vi "Take and analyse picture.vi"(0 "Training image on/off":bool, 2 "Session Out in":T3, 3 "Refnum in":T1, 5 "error in (no error)":errorcluster) -> (9 "error out":errorcluster, 10 "output cluster":T2, 14 "Insect-data-array (out of range removed)":dbl[][](array[numeric]), 15 "Initial number of insects":i32, 16 "Number of objects":i32, 17 "Session Out out":T3, 18 "Tegne cirkel array":dbl[][](array[numeric]), 19 "Black image error":bool)   [LabVIEW 2022 SP3]
doc: "Collects an image and runs it throu the vision asistent. Then transforms output data to sutible outlets and formats."
uses:
  <vilib>/userdefined/High Color/IMAQdx.ctl
  <vilib>/vision/Image Controls.llb/IMAQ Image.ctl
  <vilib>/vision/NI_Vision_Development_Module.lvlib
  <vilib>/vision/driver/NI_Vision_Acquisition_Software.lvlib
panel:
  out "Camera feed":T1(plugin-control)
  in  "Boolean":bool
  out "Image from vision assistant 2":T1(plugin-control)
  out "T_and_A Stoped":bool
  out "Match Score (Color Matching 1)":i32[](array[numeric])
  out "Objects after sorting":string[][](array[string])
  out "Image from vision assistant":T1(plugin-control)
  in  "Stop program":bool
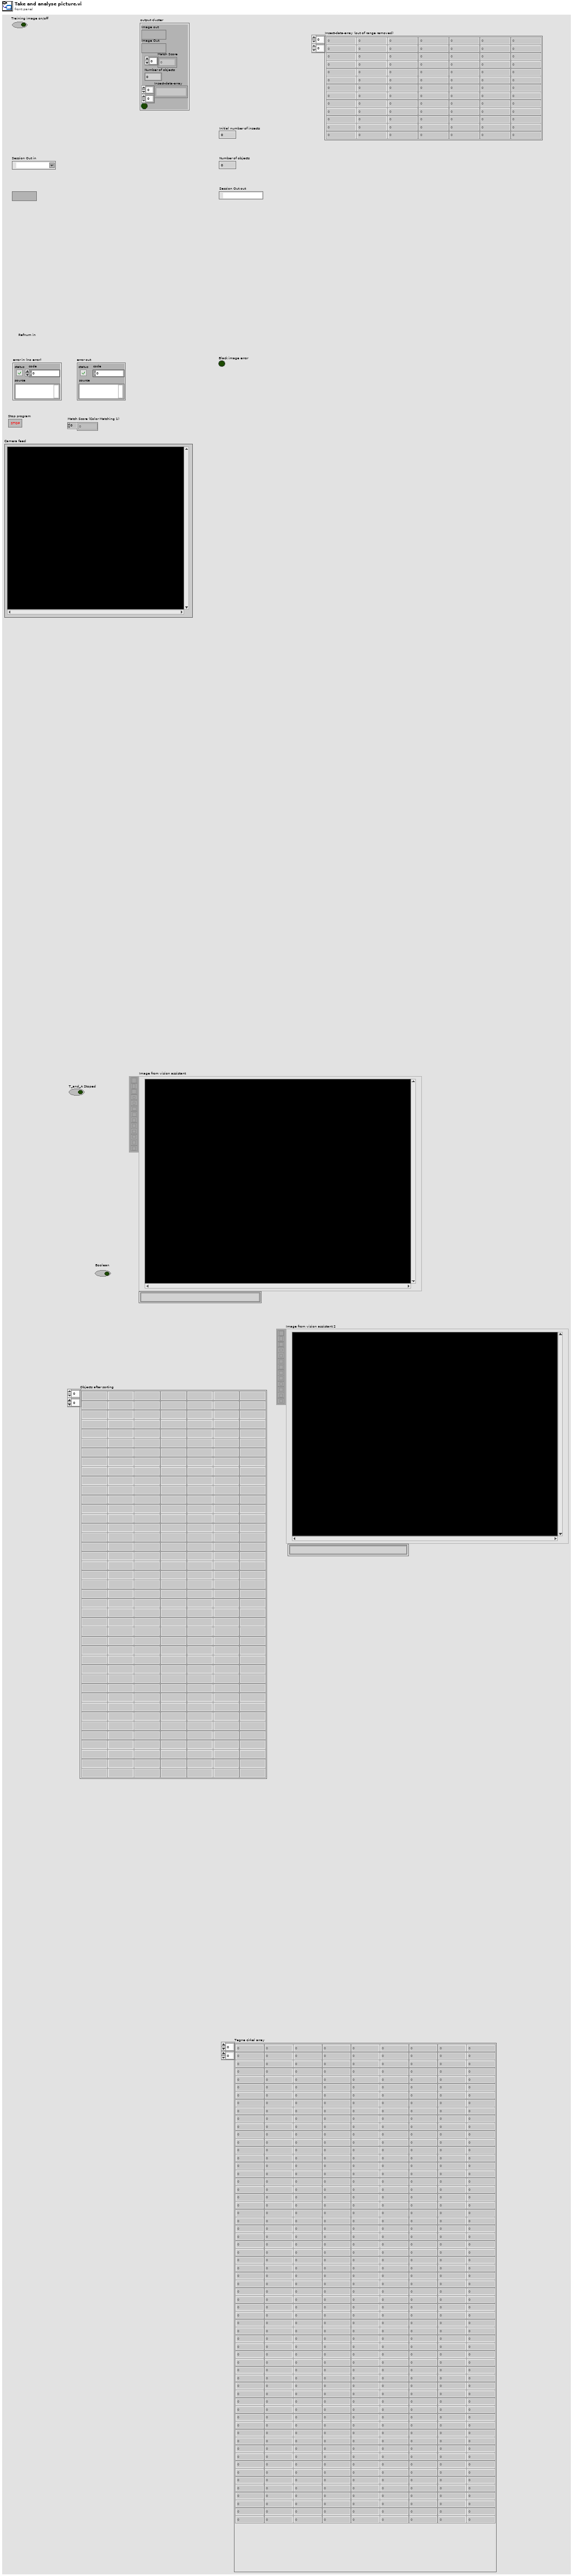
[diagram p1: front panel]
types:
  T1 = typedef "IMAQ Image.ctl" = refnum<image>
  T2 = cluster{"Image out":T1, "Image Out":T1, "Match Score":i32[], "Number of objects":i32, "Insect-data-array":string[][], bool}
  T3 = typedef "IMAQdx.ctl" = refnum<k21>
  T4 = cluster{"Measurement Parameter":i32, "Range Lower Value":dbl, "Range Upper Value":dbl, "Range":bool, "Measurement Type":bool}[]
  T5 = cluster{"Image out":T1, "Image Out":T1, "Match Score (Color Matching 1)":i32[], "Number of objects":i32, "Insect-data-array":string[][], bool}
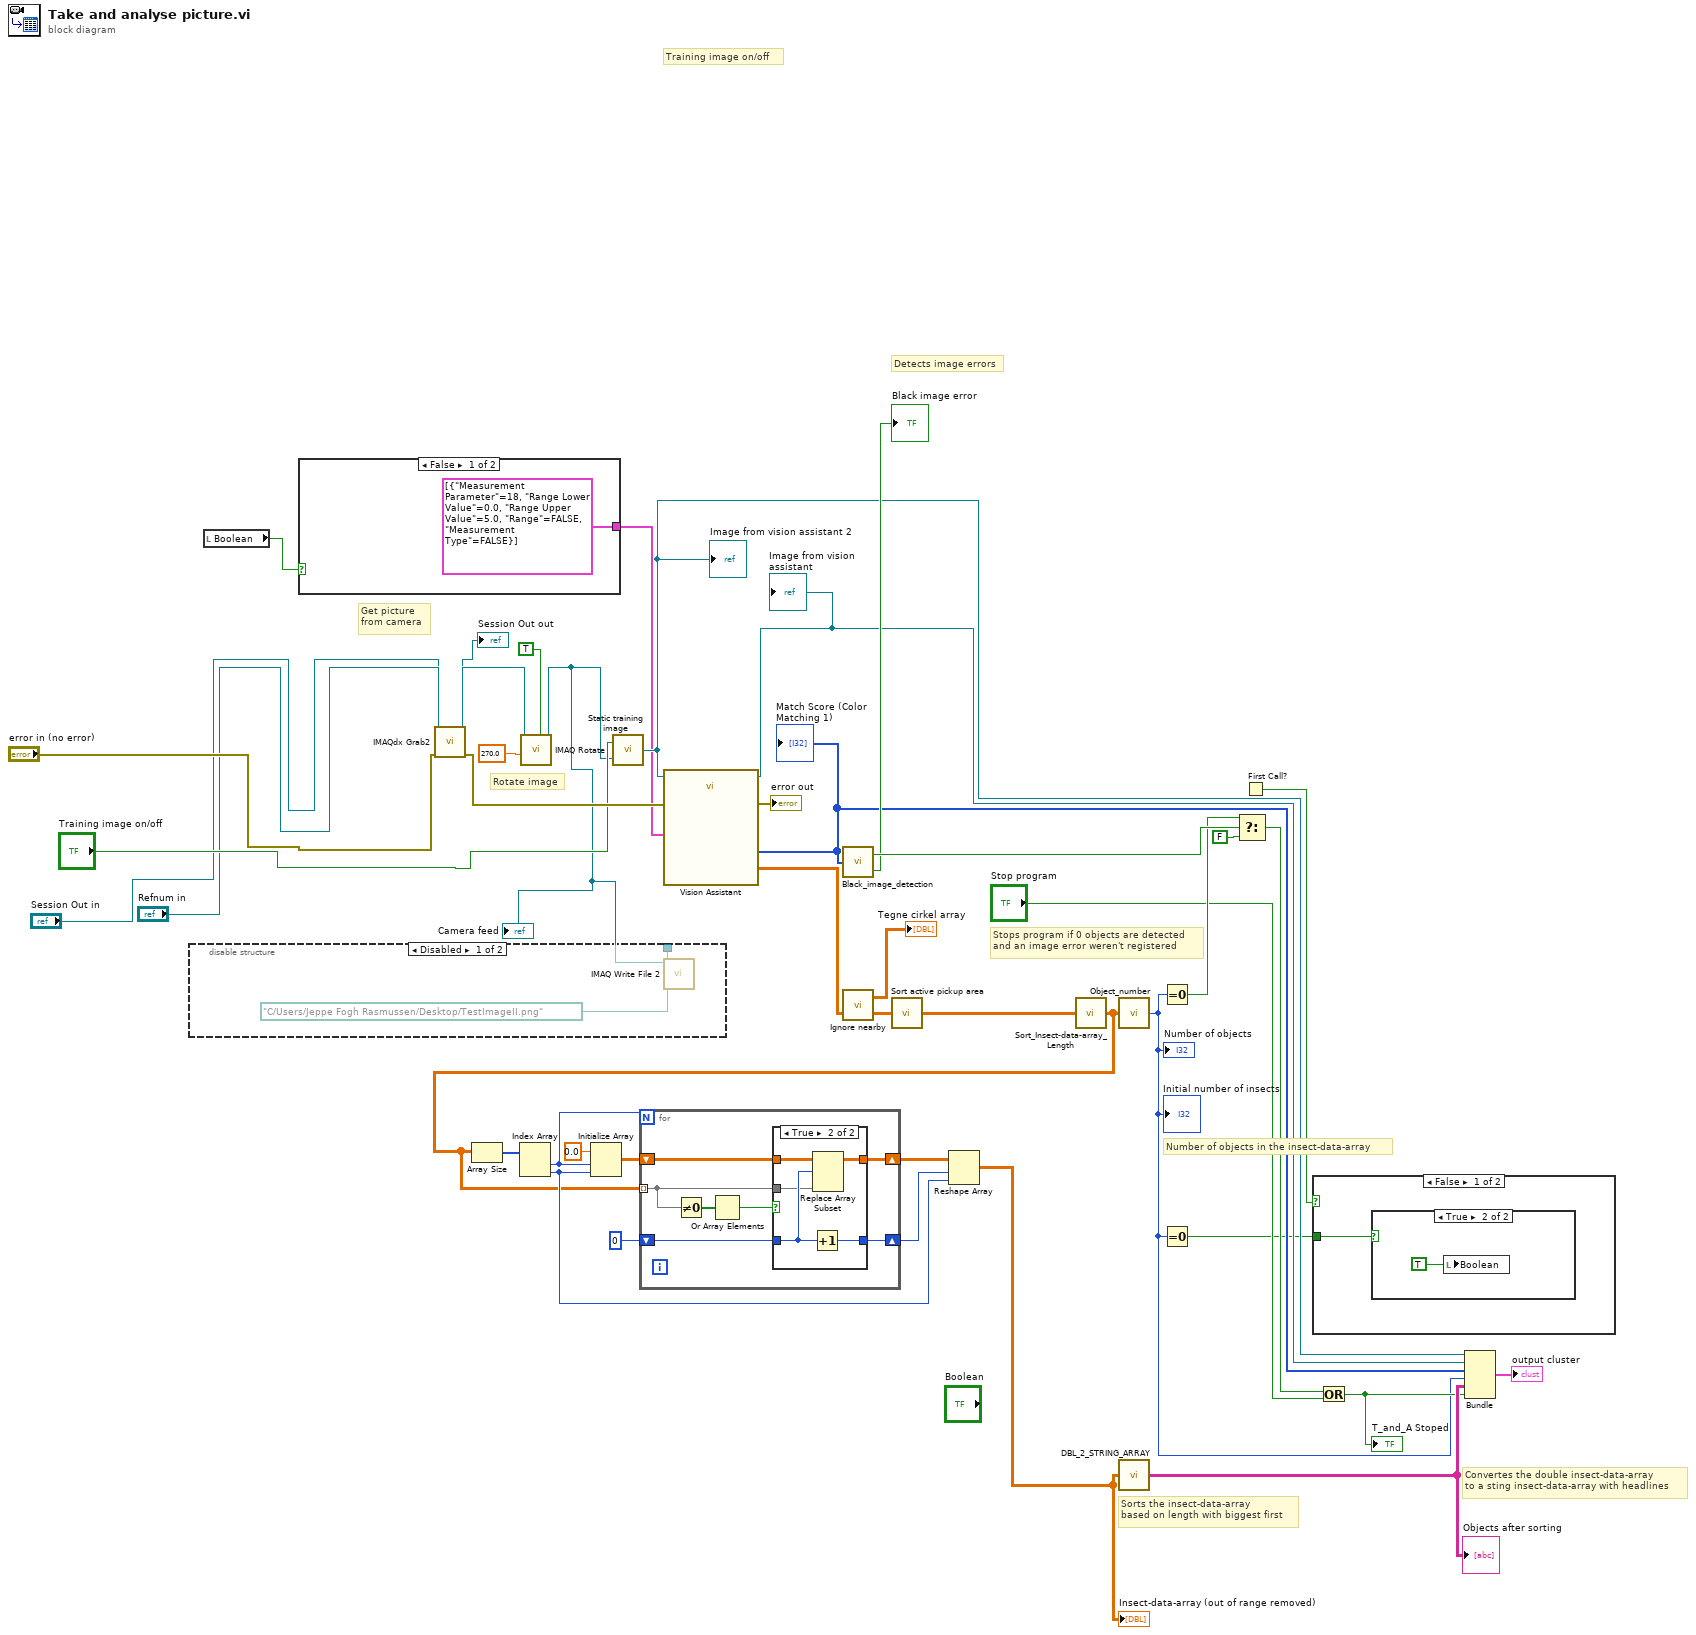
[diagram p0: block diagram]
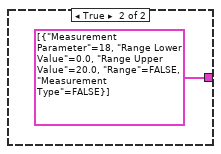
[diagram p4: hidden frame]
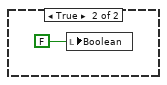
[diagram p6: hidden frame]
diagram:
  # "Detects image errors"
  # "Stops program if 0 objects are detected \nand an image error weren't registered"
  # "Number of objects in the insect-data-array"
  # "Convertes the double insect-data-array\nto a sting insect-data-array with headlines"
  # "Get picture \nfrom camera"
  # "Rotate image"
  # "Training image on/off"
  # "Sorts the insect-data-array\nbased on length with biggest first"
  n1 = local read "Boolean"() -> (w18:bool)
  n2 = case shown="False" w18 {
    tunnel: [T4 [{"Measurement Parameter"=18, "Range Lower Value"=0.0, "Range Upper Value"=5.0, "Range"=FALSE, "Measurement Type"=FALSE}] ("Selection Values (Particle Filter 2)") T4 [{"Measurement Parameter"=18, "Range Lower Value"=0.0, "Range Upper Value"=20.0, "Range"=FALSE, "Measurement Type"=FALSE}] ("Selection Values (Particle Filter 2)")] -> w20
    frame False {
    }
    frame True {
    }
  }
  n3 = call <vilib>:"IMAQdx Grab2.vi"("error in"="error in (no error)", "Image In"="Refnum in", "Session In"="Session Out in") -> ("error out"=w30:errorcluster, "Image Out"=w37:T1, "Session Out"=→"Session Out out":T3)  [unwired: 5 in, 1 out]
  n4 = call "IMAQ Rotate"("Maintain Size"=TRUE, "Angle (degrees)"=sgl 270.0, "Image Src"=w37) -> ("Image Dst Out"=w1:T1)  [unwired: 7 in, 1 out]
  "Camera feed" <- w1
  n5 = disable-structure shown="Disabled" {
    disable-tunnel: w1 -> [w46 _]
    frame Disabled {
      n6 = call-poly "IMAQ Write File 2"("File Path"=path "C:/Users/Jeppe Fogh Rasmussen/Desktop/TestImageII.png", "Image"=w46) -> ()  [unwired: 8 in, 2 out]
    }
    frame Enabled {
    }
  }
  n7 = call "Static training image.vi"("Image in"=w1, "Training image on/off"="Training image on/off") -> ("Image out"=w31:T1)
  "Image from vision assistant 2" <- w31
  n8 = call "Vision Assistant"("Image In"=w31, "Selection Values (Particle Filter 2)"=w20, "error in"=w30) -> ("Image Out"=w29:T1, "Particle Measurements (Real-World) (Particle Analysis 1)"=w25:dbl[][], "Match Score (Color Matching 1)"=w28:i32[], "error out"=→"error out":errorcluster)  [unwired: 21 in]
  "Image from vision assistant" <- w29
  "Match Score (Color Matching 1)" <- w28
  n9 = call "Black_image_detection.vi"("Match score"=w28) -> ("Black image error"=w42:bool, "Image taken without error"=→"Black image error":bool)
  n10 = call "Ignore nearby.vi"("Particle Measurements (Real-World) (Particle Analysis 1)"=w25) -> ("s? t:f"=w21:dbl[][], "appended array"=→"Tegne cirkel array":dbl[][])  [unwired: 1 in]
  n11 = call "Sort active pickup area.vi"("Insect-data-array"=w21) -> ("Insect-data-array (out of range removed)"=w26:dbl[][])  [unwired: 2 in]
  n12 = call "Sort_Insect-data-array_Length.vi"("Insect-data-array"=w26) -> ("Insect-data-array (sorted-length)"=w5:dbl[][])
  n13 = Array Size(array=w5) -> (size(s)=w12:i32[])
  n14 = Index Array(array=w12) -> (element #1=w10:i32, element #2=w6:i32)  [unwired: 2 in]
  n15 = Initialize Array(0.0, w10, w6) -> (w11:dbl[][])
  n16 = for {
    N: w10 -> [_]
    shift-right: [w53] -> w7
    shift-left: w11 -> [w52]
    shift-right: [w50] -> w8
    shift-left: 0 -> [w51]
    tunnel: w5 -> [w47] mode=indexing
    n17 = Not Equal To 0?(x=w47) -> (x != 0?=w49:bool[])
    n18 = Or Array Elements(Boolean array=w49) -> (logical OR=w48:bool)
    n19 = case shown="True" w48 {
      tunnel: w52 -> [w55 w60]
      tunnel: [w55 w59] -> w53
      tunnel: w51 -> [w54 w57]
      tunnel: [w54 w58] -> w50
      tunnel: w47 -> [_ w56]
      frame False {
      }
      frame True {
        n20 = Increment(x=w57) -> (x+1=w58:i32)
        n21 = Replace Array Subset(array=w60, new element=w56, index (row)=w57) -> (w59:dbl[][])  [unwired: 1 in]
      }
    }
  }
  n22 = Reshape Array(w7, w8, w6) -> (w4:dbl[][])
  "Insect-data-array (out of range removed)" <- w4
  n23 = call "Object_number.vi"("Insect-data-array"=w5) -> ("Number of objects"=w19:i32)
  "Initial number of insects" <- w19
  "Number of objects" <- w19
  n24 = call "DBL_2_STRING_ARRAY.vi"("Insect-data-array"=w4) -> ("Insect-data-array"=w35:string[][])
  "Objects after sorting" <- w35
  n25 = Equal To 0?(x=w19) -> (x = 0?=w39:bool)
  n26 = Equal To 0?(x=w19) -> (x = 0?=w23:bool)
  n27 = Select(t=w39, s=w42, f=FALSE) -> (s? t:f=w40:bool)
  n28 = First Call?() -> (First Call?: T/F=w24:bool)
  n29 = case shown="False" w24 {
    tunnel: w23 -> [w61 _]
    frame False {
      n30 = case shown="True" w61 {
        frame False {
        }
        frame True {
          n31 = local write "Boolean"(TRUE) -> ()
        }
      }
    }
    frame True {
      n32 = local write "Boolean"(FALSE) -> ()
    }
  }
  n33 = Or(x=w40, y="Stop program") -> (x .or. y?=w33:bool)
  "T_and_A Stoped" <- w33
  n34 = Bundle("Image out"=w31, "Image Out"=w29, "Match Score (Color Matching 1)"=w28, "Number of objects"=w19, "Insect-data-array"=w35, w33) -> (→"output cluster":T5)  [unwired: 1 in]
